vi "Periodic Tasks.vi"(8 "error in":errorcluster) -> ()   [LabVIEW 2018]
doc: "This VI runs in parallel to other tasks. It can contain as many user-defined periodic loops as you need. These can carry out PID or other sorts of timed response."
uses:
  <vilib>/Rock Robotics/WPI/Solenoid/WPI_SolenoidValue.ctl
  <vilib>/Rock Robotics/WPI/Relay/WPI_RelayValue.ctl
  <vilib>/Rock Robotics/Network Tables/NT Read Boolean.vi
  Globals.vi
  <vilib>/Rock Robotics/Network Tables/NT Write String.vi
  <vilib>/Rock Robotics/WPI/Solenoid/WPI_SolenoidSetEnum.vi
  navx-mxp/labview/navX Library v2/navX Library v2.lvlib
panel:
  out "navX axes":T1
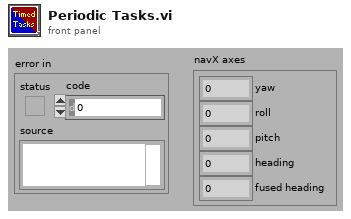
[diagram p1: front panel]
types:
  T1 = cluster{"yaw":dbl, "roll":dbl, "pitch":dbl, "heading":dbl, "fused heading":dbl}
  T2 = typedef "navX Library v2.lvlib/Z900_navX_DeviceTypeDef.ctl" = cluster{"Interface":cluster{"Protocol":T3, "Update Rate (4Hz-100Hz)":u8, "navX Open TypeDef":variant}, "Notify Packet":refnum<notifier>, "Loop VI Refnum":refnum<vi>, "Ready to Close Occurrence Refnum":refnum<k4>}
  T3 = typedef "navX Library v2.lvlib/Z900_navX_ProtocolTypeDef.ctl" = enum16{"SERIAL", "I2C", "SPI"}
  T4 = typedef "WPI_AnalogChannelDevRef.ctl" = cluster{"DevStatus":errorcluster, "Analog Channel":T5}
  T5 = typedef "FPGA_AIChannel.ctl" = enum8{"AI 0", "AI 1", "AI 2", "AI 3", "AI MXP 0", "AI MXP 1", "AI MXP 2", "AI MXP 3", "Invalid"}
  T6 = typedef "WPI_MotorControlDeviceRef.ctl" = cluster{"DeviceStatus":errorcluster, "Type":T7, "PWM":cluster{"PWM Channel":T8, "DeadBand":T9}, "CAN":cluster{"Device Number":u8, "SetOutput VI Ref":variant, "GetOutput VI Ref":variant, "Enable VI Ref":variant, "Disable VI Ref":variant, "Data":variant}, "Invert":bool, "DIO PWM":cluster{"PWM \"Enable\" Channel":T8, "DIOChannel":T10, "PWM Rate":dbl}}
  T7 = typedef "WPI_MotorControlType.ctl" = enum16{"PWM", "CAN", "DIO PWM"}
  T8 = typedef "FPGA_DIOPWMChannel.ctl" = enum8{"PWM 0", "PWM 1", "PWM 2", "PWM 3", "PWM 4", "PWM 5", "PWM 6", "PWM 7", "PWM 8", "PWM 9", "PWM MXP 0", "PWM MXP 1", "PWM MXP 2", "PWM MXP 3", "PWM MXP 4", "PWM MXP 5", "PWM MXP 6", "PWM MXP 7", "PWM MXP 8", "PWM MXP 9", "Invalid"}
  T9 = typedef "WPI_PWMDeadband.ctl" = cluster{"Name":string, "maxPositivePwm":i32, "minPositivePwm":i32, "centerPwm":i32, "maxNegativePwm":i32, "minNegativePwm":i32, "angularRange":u16}
  T10 = typedef "FPGA_DIOChannel.ctl" = enum8{"DIO 0", "DIO 1", "DIO 2", "DIO 3", "DIO 4", "DIO 5", "DIO 6", "DIO 7", "DIO 8", "DIO 9", "DIO MXP 0", "DIO MXP 1", "DIO MXP 2", "DIO MXP 3", "DIO MXP 4", "DIO MXP 5", "DIO MXP 6", "DIO MXP 7", "DIO MXP 8", "DIO MXP 9", "DIO MXP 10", "DIO MXP 11", "DIO MXP 12", "DIO MXP 13", "DIO MXP 14", "DIO MXP 15", "SPI Port CS1", "SPI Port CS2", "SPI Port CS3", "SPI Port MISO", "SPI Port MOSI", "Invalid"}
  T11 = typedef "WPI_EncoderDevRef.ctl" = cluster{"DevStatus":errorcluster, "EncoderIndex":T12, "CounterIndex":T13, "DistancePerCount":dbl, "Decoding Type":T14}
  T12 = typedef "FPGA_EncoderIdx.ctl" = enum8{"Enc 0", "Enc 1", "Enc 2", "Enc 3", "Enc 4", "Enc 5", "Enc 6", "Enc 7", "Invalid"}
  T13 = typedef "FPGA_CounterCtrSystemIndex.ctl" = enum8{"Ctr 0", "Ctr 1", "Ctr 2", "Ctr 3", "Ctr 4", "Ctr 5", "Ctr 6", "Ctr 7", "Invalid"}
  T14 = typedef "WPI_EncoderType.ctl" = enum16{"1x", "2x", "4x"}
  T15 = typedef "WPI_RelayDevRef.ctl" = cluster{"DevStatus":errorcluster, "Relay Channel":T16, "Relay Direction":T17}
  T16 = typedef "FPGA_DIORelayChannel.ctl" = enum8{"Relay 0", "Relay 1", "Relay 2", "Relay 3", "Invalid"}
  T17 = typedef "WPI_RelayDirection.ctl" = enum16{"Both directions", "Forward only", "Reverse only"}
  T18 = typedef "WPI_SolenoidDevRef.ctl" = cluster{"DevStatus":errorcluster, "Pneumatics Control Module":u8, "Forward Solenoid Channel":T19, "Reverse Solenoid Channel":T19}
  T19 = typedef "WPI_SolenoidChannel.ctl" = enum8{"Solenoid 0", "Solenoid 1", "Solenoid 2", "Solenoid 3", "Solenoid 4", "Solenoid 5", "Solenoid 6", "Solenoid 7", "Invalid"}
  T20 = typedef "WPI_SolenoidValue.ctl" = enum16{"Off", "On", "Forward", "Reverse"}
  T21 = typedef "WPI_RelayValue.ctl" = enum16{"Off", "On", "Forward", "Reverse"}
  T22 = cluster{"Yaw":dbl, "Roll":dbl, "Pitch":dbl, "Heading":dbl, "Fused Heading":dbl}
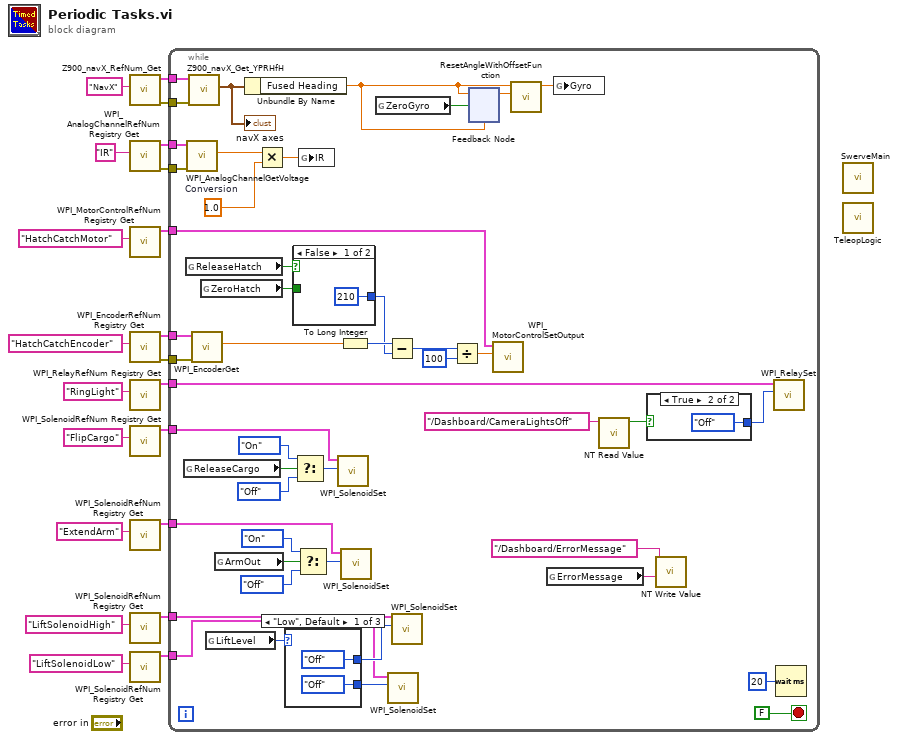
[diagram p0: block diagram]
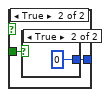
[diagram p2: hidden frame]
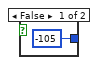
[diagram p3: hidden frame]
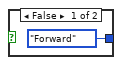
[diagram p4: hidden frame]
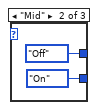
[diagram p5: hidden frame]
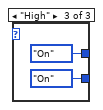
[diagram p6: hidden frame]
diagram:
  n1 = call "Z900_navX_RefNum_Get.vi"("refnum name"="NavX") -> ("error out"=w4:errorcluster, "navX Device"=w20:T2)  [unwired: 9 in]
  n2 = call <vilib>:"WPI_AnalogChannelRefNum Registry Get.vi"("refnum name"="IR") -> ("error out"=w18:errorcluster, "AIDeviceRef"=w1:T4)  [unwired: 9 in]
  n3 = call <vilib>:"WPI_MotorControlRefNum Registry Get.vi"("refnum name"="HatchCatchMotor") -> ("MotorControlDevRef"=w17:T6)  [unwired: 9 in, 1 out]
  n4 = call <vilib>:"WPI_EncoderRefNum Registry Get.vi"("refnum name"="HatchCatchEncoder") -> ("error out"=w9:errorcluster, "EncoderDevRef"=w10:T11)  [unwired: 9 in]
  n5 = call <vilib>:"WPI_RelayRefNum Registry Get.vi"("refnum name"="RingLight") -> ("RelayDevRef"=w2:T15)  [unwired: 9 in, 1 out]
  n6 = call <vilib>:"WPI_SolenoidRefNum Registry Get.vi"("refnum name"="FlipCargo") -> ("SolenoidDevRef"=w6:T18)  [unwired: 9 in, 1 out]
  n7 = call <vilib>:"WPI_SolenoidRefNum Registry Get.vi"("refnum name"="ExtendArm") -> ("SolenoidDevRef"=w5:T18)  [unwired: 9 in, 1 out]
  n8 = call <vilib>:"WPI_SolenoidRefNum Registry Get.vi"("refnum name"="LiftSolenoidHigh") -> ("SolenoidDevRef"=w16:T18)  [unwired: 9 in, 1 out]
  n9 = call <vilib>:"WPI_SolenoidRefNum Registry Get.vi"("refnum name"="LiftSolenoidLow") -> ("SolenoidDevRef"=w15:T18)  [unwired: 9 in, 1 out]
  n10 = while {
    tunnel: w20 -> [w61]
    tunnel: w1 -> [w60]
    tunnel: w18 -> [w58]
    tunnel: w17 -> [w34]
    tunnel: w16 -> [w52]
    tunnel: w15 -> [w53]
    tunnel: w10 -> [w51]
    tunnel: w9 -> [w50]
    tunnel: w6 -> [w42]
    tunnel: w5 -> [w37]
    tunnel: w4 -> [w35]
    tunnel: w2 -> [w30]
    stop <- FALSE stop-if-true
    w57 = 1.0  # Conversion
    n11 = global read "Globals.vi" "ReleaseCargo"() -> (w46:bool)
    n12 = global read "Globals.vi" "ReleaseHatch"() -> (w29:bool)
    n13 = call <vilib>:"WPI_AnalogChannelGetVoltage.vi"("error in (no error)"=w58, "AIDeviceRef"=w60) -> ("Voltage"=w59:dbl)  [unwired: 7 in, 2 out]
    n14 = call "Z900_navX_Get_YPRHfH.vi"("error in (no error)"=w35, "navX Device"=w61) -> ("YRPHfH"=w64:T22)  [unwired: 6 in, 3 out]
    "navX axes" <- w64
    n15 = call <vilib>:"WPI_EncoderGet.vi"("error in (no error)"=w50, "EncoderDevRef"=w51) -> ("Distance"=w27:dbl)  [unwired: 4 in, 5 out]
    n16 = global read "Globals.vi" "ZeroHatch"() -> (w28:bool)
    n17 = global read "Globals.vi" "LiftLevel"() -> (w56:enum16{"Low", "Mid", "High"})
    n18 = global read "Globals.vi" "ArmOut"() -> (w41:bool)
    n19 = Unbundle By Name(w64) -> ("Fused Heading"=w36:dbl)
    n20 = Multiply(x=w59, y=w57) -> (x*y=w49:dbl)
    n21 = case shown="\"Low\", Default" w56 {
      tunnel: [WPI_SolenoidValue."Off" ("Value") WPI_SolenoidValue."Off" ("Value") WPI_SolenoidValue."On" ("Value")] -> w55
      tunnel: [WPI_SolenoidValue."Off" ("Value") WPI_SolenoidValue."On" ("Value") WPI_SolenoidValue."On" ("Value")] -> w54
      frame "Low", Default {
      }
      frame "Mid" {
      }
      frame "High" {
      }
    }
    n22 = case shown="False" w29 {
      tunnel: w28 -> [_ w70]
      tunnel: [210 w69] -> w25
      frame False {
      }
      frame True {
        n23 = case shown="True" w70 {
          tunnel: [-105 0] -> w69
          frame False {
          }
          frame True {
          }
        }
      }
    }
    n24 = Select(t=WPI_SolenoidValue."On" ("Value"), s=w46, f=WPI_SolenoidValue."Off") -> (s? t:f=w43:T20)
    n25 = Select(t=WPI_SolenoidValue."On" ("Value"), s=w41, f=WPI_SolenoidValue."Off") -> (s? t:f=w38:T20)
    n26 = global write "Globals.vi" "IR"(w49) -> ()
    n27 = call-poly <vilib>:"WPI_SolenoidSet.vi"("Value"=w43, "SolenoidDevRef"=w42) -> ()  [unwired: 8 in, 2 out]
    n28 = To Long Integer(number=w27) -> (32bit integer=w26:i32)
    n29 = call-poly <vilib>:"WPI_SolenoidSet.vi"("Value"=w38, "SolenoidDevRef"=w37) -> ()  [unwired: 8 in, 2 out]
    n30 = global read "Globals.vi" "ZeroGyro"() -> (w62:bool)
    n31 = Subtract(x=w26, y=w25) -> (x-y=w24:i32)
    n32 = call-poly <vilib>:"WPI_SolenoidSet.vi"("Value"=w54, "SolenoidDevRef"=w53) -> ()  [unwired: 8 in, 2 out]
    n33 = call-poly <vilib>:"WPI_SolenoidSet.vi"("Value"=w55, "SolenoidDevRef"=w52) -> ()  [unwired: 8 in, 2 out]
    n34 = Divide(x=w24, y=100) -> (x/y=w22:dbl)
    n35 = feedback-in #1(w36, w62) -> ()
    n36 = feedback #1(w36) -> (w65:dbl)
    n37 = call <vilib>:"WPI_MotorControlSetOutput.vi"("Output"=w22, "MotorControlDevRef"=w34) -> ()  [unwired: 7 in, 3 out]
    n38 = call "ResetAngleWithOffsetFunction.vi"("Offset"=w65, "AngleInput"=w36) -> ("AngleOutput"=w63:dbl)  [unwired: 9 in]
    n39 = global read "Globals.vi" "ErrorMessage"() -> (w48:string)
    n40 = global write "Globals.vi" "Gyro"(w63) -> ()
    n41 = call-poly <vilib>:"NT Read Value.vi"("Name"="/Dashboard/CameraLightsOff") -> ("Boolean"=w32:bool)  [unwired: 9 in, 1 out]
    n42 = case shown="True" w32 {
      tunnel: [WPI_RelayValue."Forward" ("RelayValue") WPI_RelayValue."Off" ("RelayValue")] -> w31
      frame False {
      }
      frame True {
      }
    }
    n43 = call-poly <vilib>:"NT Write Value.vi"("String"=w48, "Name"="/Dashboard/ErrorMessage") -> ()  [unwired: 9 in, 1 out]
    n44 = call <vilib>:"WPI_RelaySet.vi"("RelayValue"=w31, "RelayDevRef"=w30) -> ()  [unwired: 8 in, 2 out]
    n45 = Wait (ms)(milliseconds to wait=u32 20) -> ()  [unwired: 1 out]
  }
  n46 = call "SwerveMain.vi"() -> ()  [unwired: 12 in]
  n47 = call "TeleopLogic.vi"() -> ()  [unwired: 12 in]
